vi "read_bit.vi"(10 "Min time SCL low":u32, 11 "Min Time SCL high":u32) -> (3 "Data bit":bool)   [LabVIEW 2019]
uses:
  <vilib>/rvi/eio/common/nirviEmuTemplateMethod_errors.vi
  <vilib>/eio/EIOMethodNode/EIOMethodNode.xnode
  <vilib>/eio/EIONode/EIONode.xnode
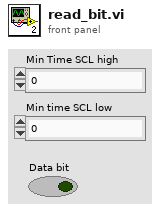
[diagram p1: front panel]
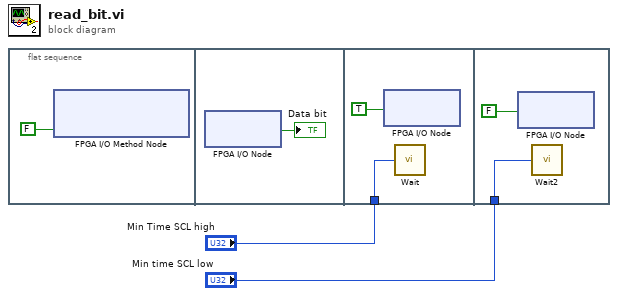
[diagram p0: block diagram]
diagram:
  n1 = flat-sequence {
    tunnel: "Min Time SCL high" -> [w5]
    tunnel: "Min time SCL low" -> [w7]
    frame #0 {
      n2 = xnode "FPGA I/O Method Node"("Enable"=FALSE ("Digital Enable")) -> ()  [unwired: 1 in, 1 out]
    }
    frame #1 {
      n3 = xnode "FPGA I/O Node"() -> ("SDA"=→"Data bit":bool)  [unwired: 1 in, 1 out]
    }
    frame #2 {
      n4 = xnode "FPGA I/O Node"("SCL"=TRUE ("Digital Out")) -> ()  [unwired: 1 in, 1 out]
      n5 = call "Wait"("Count(uSec)"=w5) -> ()  [unwired: 1 out]
    }
    frame #3 {
      n6 = xnode "FPGA I/O Node"("SCL"=FALSE ("Digital Out")) -> ()  [unwired: 1 in, 1 out]
      n7 = call "Wait2"("Count(uSec)"=w7) -> ()  [unwired: 1 out]
    }
  }
